vi "Temp Ctrl Path.vi"() -> (3 "appended path":path)   [LabVIEW 2023]
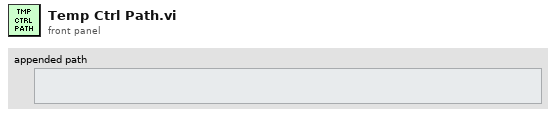
[diagram p1: front panel]
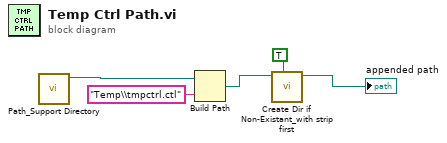
[diagram p0: block diagram]
diagram:
  n1 = call "Path_Support Directory.vi"() -> ("Support Directory"=w5:path)  [unwired: 11 in]
  n2 = Build Path(base path=w5, name or relative path="Temp\\tmpctrl.ctl") -> (appended path=w2:path)
  n3 = call "Create Dir if Non-Existant_with strip first.vi"("Strip Path First [F]"=TRUE, "Directory Path"=w2) -> ("dup Directory Path"=→"appended path":path)  [unwired: 7 in, 2 out]
